vi "SLL DE Read DAQ Engine Parameters form INI File.vi"(8 "error in (no error)":errorcluster) -> (0 "error out":errorcluster)   [LabVIEW 2013]
uses:
  Controls/SLL DE DAQ Engine Parameters.ctl
  Controls/SLL DE List of Analog Outputs.ctl
  Controls/SLL DE List of Digital Outputs.ctl
  Controls/SLL DE List of Analog Inputs.ctl
  Controls/SLL DE List of AI Channel Type.ctl
  Controls/SLL DE DAQ Parameters LV2Global Options.ctl
  <vilib>/Utility/config.llb/NI_LVConfig.lvlib
panel:
  in  "DAQ Engine":T1={"Enable Engines"={"AI Enable"=TRUE, "AO Enable"=TRUE, "DI Enable"=TRUE, "DO Enable"=TRUE}, "DAQ Control Type"={"Analog Input"=enum."Finite", "Analog Output"=enum."Finite", "Digital Input"=enum."Finite", "Digital Output"=enum."Finite"}, "DAQ Parameters"={"AI Sampling Rate (Samples/Sec)"=1000.0, "MvgAVG Window Size (# of Points)"=20, "Enable Filter"=TRUE, "Enable MvgAVG"=TRUE, "Circular Buffer Size (Sec)"=5.0, "AO Sampling Rate (Samples/Sec)"=1000.0, "Graph Update Rate (Samples/Sec)"=0.0, "File Logging Rate (Samples/Sec)"=500}, "AO Safe Values"=[], "DO Safe Values"=[], "DO Interconnected Lines"=[], "AI Channels Unit"=[], "Units Information"=[]}
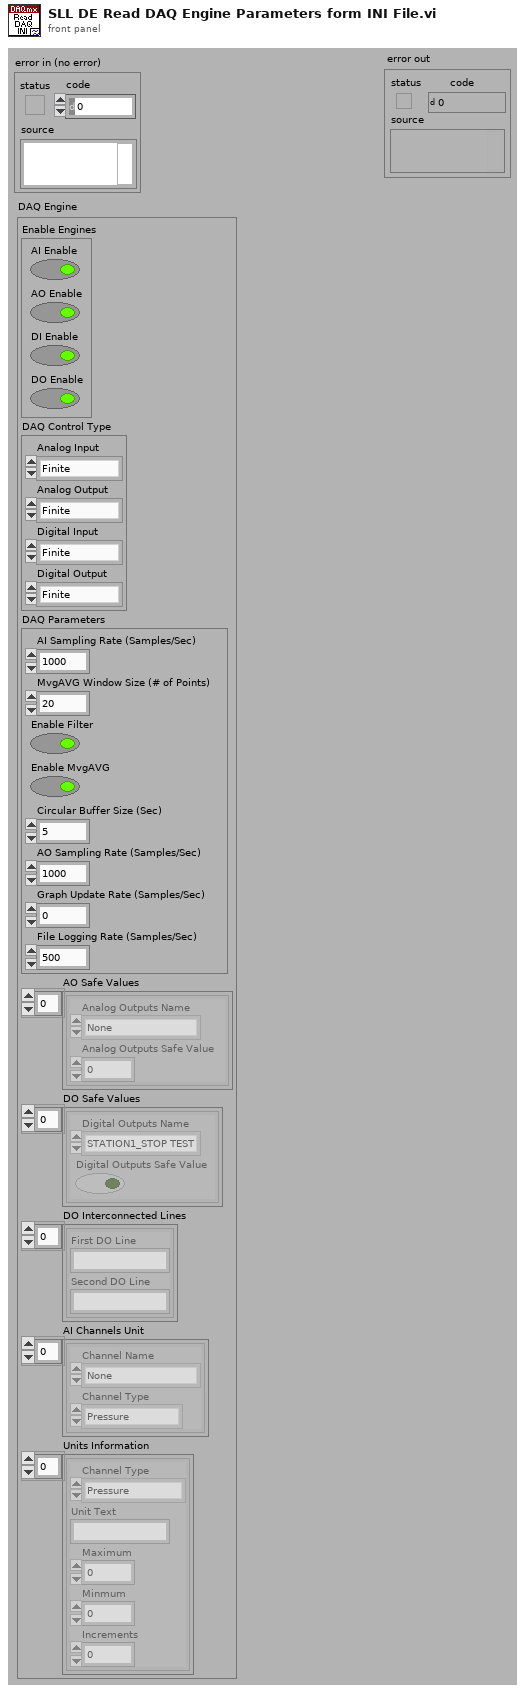
[diagram p1: front panel]
types:
  T1 = typedef "SLL DE DAQ Engine Parameters.ctl" = cluster{"Enable Engines":cluster{"AI Enable":bool, "AO Enable":bool, "DI Enable":bool, "DO Enable":bool}, "DAQ Control Type":cluster{"Analog Input":enum16{"Finite", "Continuous", "Driver"}, "Analog Output":enum16{"Finite", "Continuous", "Driver"}, "Digital Input":enum16{"Finite", "Continuous", "Driver"}, "Digital Output":enum16{"Finite", "Continuous", "Driver"}}, "DAQ Parameters":cluster{"AI Sampling Rate (Samples/Sec)":dbl, "MvgAVG Window Size (# of Points)":i32, "Enable Filter":bool, "Enable MvgAVG":bool, "Circular Buffer Size (Sec)":dbl, "AO Sampling Rate (Samples/Sec)":dbl, "Graph Update Rate (Samples/Sec)":dbl, "File Logging Rate (Samples/Sec)":i32}, "AO Safe Values":cluster{"Analog Outputs Name":T2, "Analog Outputs Safe Value":dbl}[], "DO Safe Values":cluster{"Digital Outputs Name":T3, "Digital Outputs Safe Value":bool}[], "DO Interconnected Lines":cluster{"First DO Line":string, "Second DO Line":string}[], "AI Channels Unit":cluster{"Channel Name":T4, "Channel Type":T5}[], "Units Information":cluster{"Channel Type":T5, "Unit Text":string, "Maximum":dbl, "Minmum":dbl, "Increments":dbl}[]}
  T2 = typedef "SLL DE List of Analog Outputs.ctl" = enum16{"None"}
  T3 = typedef "SLL DE List of Digital Outputs.ctl" = enum16{"STATION1_START TEST", "STATION1_STOP TEST", "STATION1_LIGHT1", "STATION1_LIGHT2", "STATION1_LIGHT3", "STATION1_SELECT_TEST", "STATION2_START TEST", "STATION2_STOP TEST", "STATION2_LIGHT1", "STATION2_LIGHT2", "STATION2_LIGHT3", "STATION2_SELECT_TEST", "STATION3_START TEST", "STATION3_STOP TEST", "STATION3_LIGHT1", "STATION3_LIGHT2", "STATION3_LIGHT3", "STATION3_SELECT_TEST", "STATION4_START TEST", "STATION4_STOP TEST", "STATION4_LIGHT1", "STATION4_LIGHT2", "STATION4_LIGHT3", "STATION4_SELECT_TEST"}
  T4 = typedef "SLL DE List of Analog Inputs.ctl" = enum16{"None"}
  T5 = typedef "SLL DE List of AI Channel Type.ctl" = enum16{"Pressure", "Flow", "Temperature", "Time Scale", "Voltage", "Current", "Frequency", "Sound", "Speed", "Torque", "Distance", "Channel Type 1", "Channel Type 2", "Channel Type 3"}
  T6 = typedef "SLL DE DAQ Parameters LV2Global Options.ctl" = enum16{"Read", "Write"}
  T7 = typedef "NI_LVConfig.lvlib/Config Data RefNum.ctl" = refnum<k1>
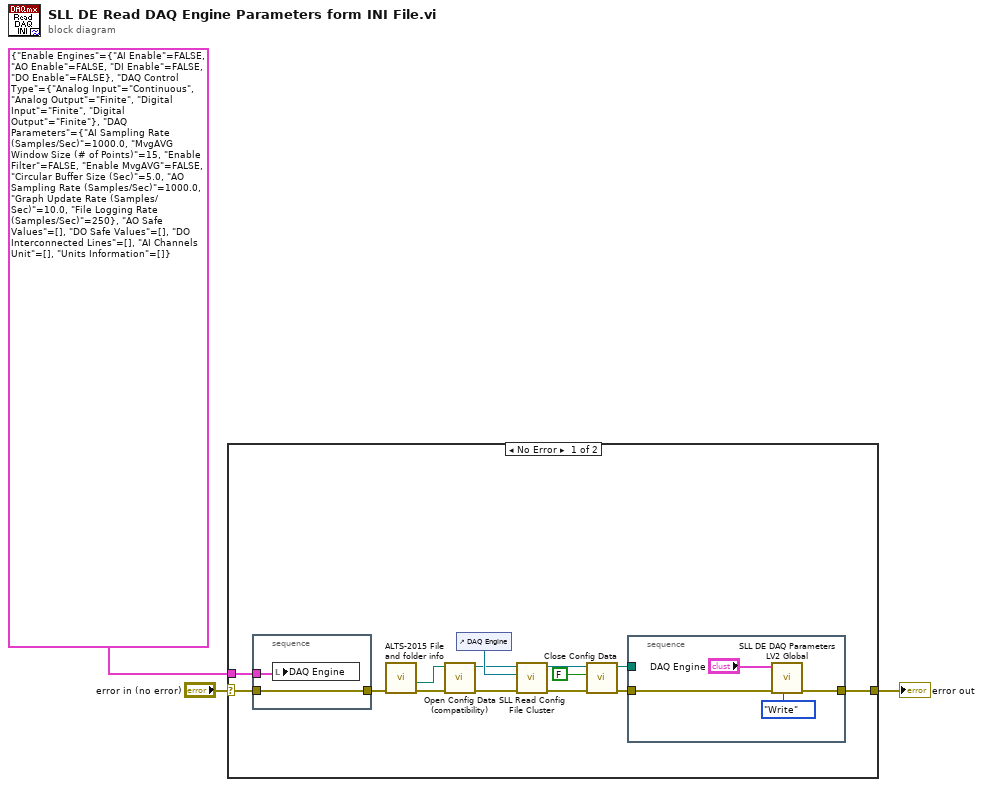
[diagram p0: block diagram]
diagram:
  n1 = case shown="No Error" "error in (no error)" {
    selector: "error in (no error)" -> [w8 w24]
    tunnel: [w10 w24] -> w2
    tunnel: T1 {"Enable Engines"={"AI Enable"=FALSE, "AO Enable"=FALSE, "DI Enable"=FALSE, "DO Enable"=FALSE}, "DAQ Control Type"={"Analog Input"=enum."Continuous", "Analog Output"=enum."Finite", "Digital Input"=enum."Finite", "Digital Output"=enum."Finite"}, "DAQ Parameters"={"AI Sampling Rate (Samples/Sec)"=1000.0, "MvgAVG Window Size (# of Points)"=15, "Enable Filter"=FALSE, "Enable MvgAVG"=FALSE, "Circular Buffer Size (Sec)"=5.0, "AO Sampling Rate (Samples/Sec)"=1000.0, "Graph Update Rate (Samples/Sec)"=10.0, "File Logging Rate (Samples/Sec)"=250}, "AO Safe Values"=[], "DO Safe Values"=[], "DO Interconnected Lines"=[], "AI Channels Unit"=[], "Units Information"=[]} ("DAQ Engine 2") -> [w7 _]
    frame No Error {
      n2 = stacked-sequence {
        tunnel: w8 -> [w19]
        tunnel: [w19] -> w5
        tunnel: w7 -> [w18]
        frame #0 {
          n3 = local write "DAQ Engine"(w18) -> ()
        }
      }
      n4 = call "ALTS-2015 File and folder info.vi"("error in (no error)"=w5) -> ("error out"=w4:errorcluster, "DAQ Engine Parameters.ini"=w6:path)  [unwired: 2 in, 7 out]
      n5 = call <vilib>:"Open Config Data (compatibility).vi"("error in (no error)"=w4, "configuration file path"=w6) -> ("error out"=w16:errorcluster, "refnum"=w15:T7)  [unwired: 7 in, 1 out]
      n6 = control-ref of="DAQ Engine"() -> (w17:refnum<vi>)
      n7 = call <userlib>:"SLL Read Config File Cluster.vi"("error in (no error)"=w16, "Config File Cluster Refnum in"=w17, "Config File Refnum in"=w15) -> ("error out"=w13:errorcluster, "Config File Refnum out"=w14:T7)  [unwired: 7 in]
      n8 = call <vilib>:"Close Config Data.vi"("error in (no error)"=w13, "write file if changed (T)"=FALSE ("write configuration file? (T)"), "refnum"=w14) -> ("error out"=w11:errorcluster, "file path"=w9:path)  [unwired: 7 in]
      n9 = stacked-sequence {
        tunnel: w11 -> [w23]
        tunnel: [w22] -> w10
        tunnel: w9 -> [_]
        frame #0 {
          n10 = call "SLL DE DAQ Parameters LV2 Global.vi"("Option"=SLL_DE_DAQ_Parameters_LV2Global_Options."Write", "Error in (no error)"=w23, "Global Info"="DAQ Engine") -> ("Error out"=w22:errorcluster)  [unwired: 7 in, 1 out]
        }
      }
    }
    frame Error {
    }
  }
  "error out" <- w2
